vi "Generated Descriptors.vi"() -> (3 "Descriptor Strings":string[](array[string]))   [LabVIEW 2020, in "Measurement Plugin Measurement Server Internal.lvlib"]
uses:
  Measurement Plugin Measurement Server Internal.lvlib
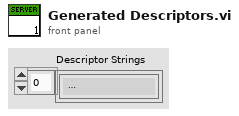
[diagram p1: front panel]
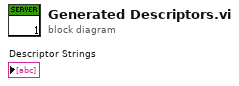
[diagram p0: block diagram]
diagram:
